vi "set encoder settings.vi"(8 "error in (no error)":errorcluster, 10 "encoder_settings":T1, 11 "id":i32) -> (0 "error out":errorcluster, 3 "function return":i32)   [LabVIEW 2012, in "libximc.lvlib"]
doc: "result_t XIMC_API set_encoder_settings (device_t id, const encoder_settings_t* encoder_settings);"
uses:
  libximc.lvlib
  libximc.dll
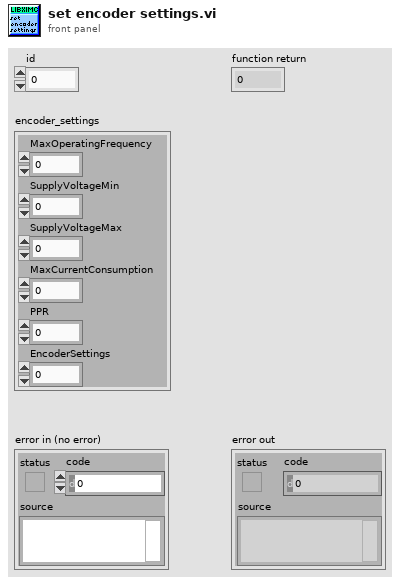
[diagram p1: front panel]
types:
  T1 = cluster{"MaxOperatingFrequency":sgl, "SupplyVoltageMin":sgl, "SupplyVoltageMax":sgl, "MaxCurrentConsumption":sgl, "PPR":u32, "EncoderSettings":u32}
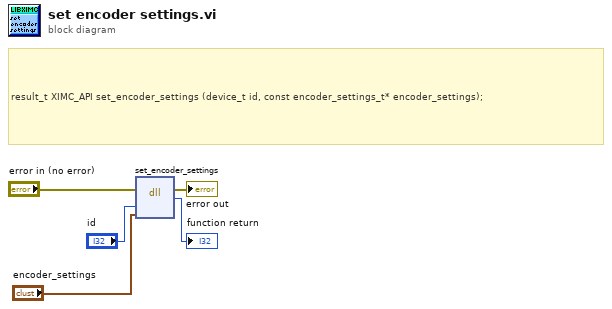
[diagram p0: block diagram]
diagram:
  # "result_t XIMC_API set_encoder_settings (device_t id, const encoder_settings_t* encoder_settings);"
  n1 = dll-call lib="C:/Users/Vasily/Att_examples/LabVIEW_example/libximc.*" fn="set_encoder_settings"(error in="error in (no error)", "id"="id", "encoder_settings"="encoder_settings") -> (error out=→"error out":errorcluster, →"function return":i32)  [unwired: 4 in, 1 out]
